vi "Draw.vi"(8 "error in (no error)":errorcluster, 10 "2D Picture in":picture, 11 "IDrawable in":refnum<class "IDrawable.lvclass">) -> (0 "error out":errorcluster, 2 "2D Picture out":picture, 3 "IDrawable out":refnum<class "IDrawable.lvclass">)   [LabVIEW 2021, in "Picture2D.lvlib" / "IDrawable.lvclass"]
uses:
  IDrawable.lvclass
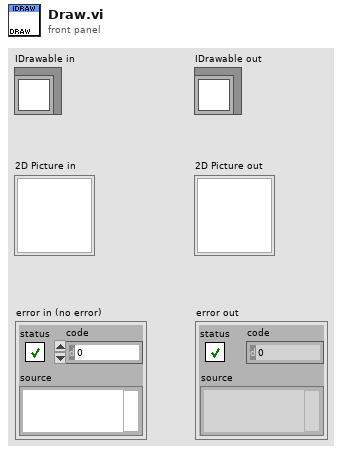
[diagram p1: front panel]
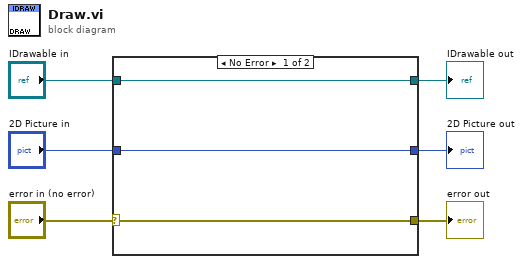
[diagram p0: block diagram]
diagram:
  n1 = case shown="No Error" "error in (no error)" {
    selector: "error in (no error)" -> [w8 w12]
    tunnel: [w8 w12] -> w5
    tunnel: [w9 w11] -> w3
    tunnel: "IDrawable in" -> [w9 w11]
    tunnel: [w7 w10] -> w1
    tunnel: "2D Picture in" -> [w7 w10]
    frame No Error {
    }
    frame Error {
    }
  }
  "error out" <- w5
  "IDrawable out" <- w3
  "2D Picture out" <- w1
